vi "Log.vi"(7 "Level":T1, 8 "Error to log":errorcluster, 9 "Source":string, 10 "Message":string, 11 "RQMHLogger in":refnum<class "Logger.lvclass">) -> (0 "Errors":errorcluster[](array[cluster]), 3 "RQMHLogger out":refnum<class "Logger.lvclass">)   [LabVIEW 2024, in "Logger.lvclass"]
uses:
  Logger.lvclass
  Logger.lvclass/Logger.ctl
  Record/LogRecord.lvclass/LogRecord.ctl
  HandleHolder/HandleHolder.lvclass/HandleHolder.ctl
  Record/LogRecord.lvclass
  LogHandle/Interface/LoggingHandle.lvclass
  HandleHolder/HandleHolder.lvclass
  Shared/Level.ctl
  Shared/LoggerShared.lvlib
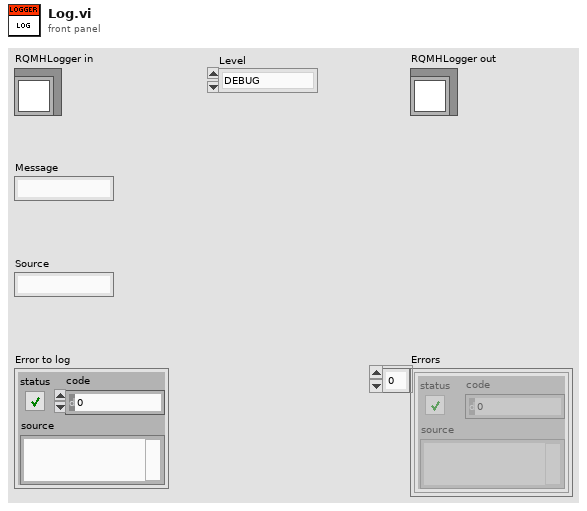
[diagram p1: front panel]
types:
  T1 = typedef "LoggerShared.lvlib/Level.ctl" = enum16{"DEBUG", "INFO", "WARNING", "ERROR", "CRITICAL"}
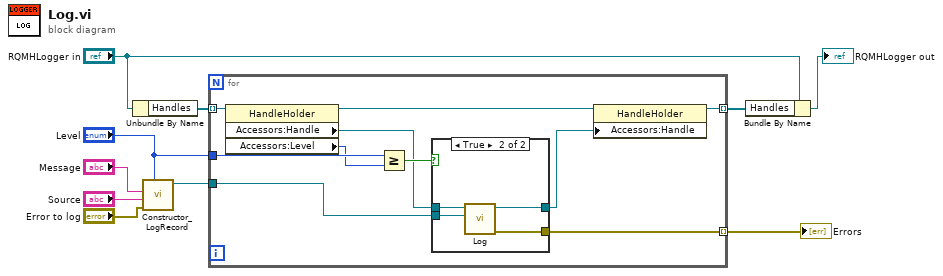
[diagram p0: block diagram]
diagram:
  n1 = Unbundle By Name("RQMHLogger in") -> ("Handles"=w10:refnum<class "HandleHolder.lvclass">[])
  n2 = call "Constructor_LogRecord.vi"("Level"="Level", "Error to log"="Error to log", "Source"="Source", "Message"="Message") -> ("LogRecord out"=w6:refnum<class "LogRecord.lvclass">)  [unwired: 7 in]
  n3 = for {
    tunnel: w10 -> [w16] mode=indexing
    tunnel: [w14] -> w7 mode=indexing
    tunnel: w6 -> [w19]
    tunnel: [w20] -> w2 mode=indexing
    tunnel: "Level" -> [w18]
    n4 = property class="HandleHolder"(reference=w16) -> (reference out=w15:refnum<class "HandleHolder.lvclass">, "Accessors:Handle"=w11:refnum<class "LoggingHandle.lvclass">, "Accessors:Level"=w12:T1)  [unwired: 1 in, 1 out]
    n5 = Greater Or Equal?(x=w18, y=w12) -> (x >= y?=w17:bool)
    n6 = case shown="True" w17 {
      tunnel: [w21 w25] -> w13
      tunnel: [_ w24] -> w20
      tunnel: w19 -> [_ w23]
      tunnel: w11 -> [w21 w22]
      frame False {
      }
      frame True {
        n7 = call-dynamic "Log.vi"("LogRecord"=w23, "LoggingHandle in"=w22) -> ("error out"=w24:errorcluster, "LoggingHandle out"=w25:refnum<class "LoggingHandle.lvclass">)  [unwired: 8 in]
      }
    }
    n8 = property class="HandleHolder"(reference=w15, "Accessors:Handle"=w13) -> (reference out=w14:refnum<class "HandleHolder.lvclass">)  [unwired: 1 in, 1 out]
  }
  "Errors" <- w2
  n9 = Bundle By Name(cluster="RQMHLogger in", "Handles"=w7) -> (→"RQMHLogger out":refnum<class "Logger.lvclass">)
